vi "Read 2D Error Bar Property Array.vi"(8 "error in (no error)":errorcluster, 11 "2D Error Bar.lvclass in":refnum<class "2D Error Bar.lvclass">) -> (0 "error out":errorcluster, 2 "2D Error Bar Property Array":T1, 3 "2D Error Bar.lvclass out":refnum<class "2D Error Bar.lvclass">)   [LabVIEW 2017, in "2D Error Bar.lvclass"]
uses:
  <vilib>/Math Plots/2D Math Plots/2D Error Bar/2D Error Bar/2D Error Bar.lvclass
  <vilib>/Math Plots/2D Math Plots/2D Error Bar/2D Error Bar/Typedef/2D Error Bar Property Array.ctl
  <vilib>/Math Plots/2D Math Plots/2D Error Bar/2D Error Bar/Typedef/2D Error Bar Property.ctl
  <vilib>/Math Plots/2D Math Plots/2D Error Bar/2D Error Bar/2D Error Bar.lvclass/2D Error Bar.ctl
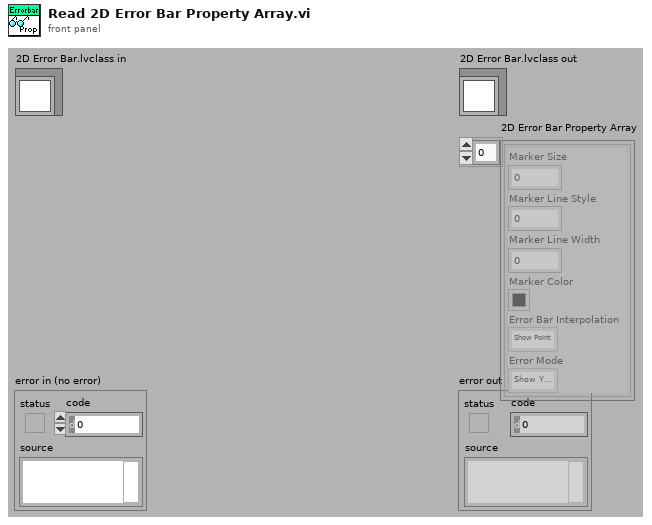
[diagram p1: front panel]
types:
  T1 = typedef "2D Error Bar.lvclass/2D Error Bar Property Array.ctl" = T2[]
  T2 = typedef "2D Error Bar.lvclass/2D Error Bar Property.ctl" = cluster{"Marker Size":dbl, "Marker Line Style":u8, "Marker Line Width":u8, "Marker Color":u32, "Error Bar Interpolation":enum16{"Show Point", "Show Line", "Show Bar"}, "Error Mode":enum16{"Show Y Error", "Show X Error", "Show Both Error"}}
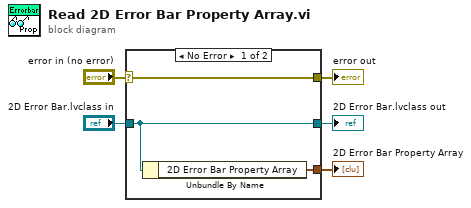
[diagram p0: block diagram]
diagram:
  n1 = case shown="No Error" "error in (no error)" {
    selector: "error in (no error)" -> [w8 w9]
    tunnel: [w8 w9] -> w4
    tunnel: [w7 w10] -> w2
    tunnel: "2D Error Bar.lvclass in" -> [w7 w10]
    tunnel: [w6 _] -> w1
    frame No Error {
      n2 = Unbundle By Name(w7) -> ("2D Error Bar Property Array"=w6:T1)
    }
    frame Error {
    }
  }
  "error out" <- w4
  "2D Error Bar.lvclass out" <- w2
  "2D Error Bar Property Array" <- w1
